vi "Auto Mode Alternate 2.vi"(1 "error in (no error)":errorcluster) -> ()   [LabVIEW 2017]
uses:
  <vilib>/Rock Robotics/WPI/Utilities/WPI_GetSetVariantRefNum.vi
  <vilib>/Rock Robotics/Network Tables/NT Write Numeric Array.vi
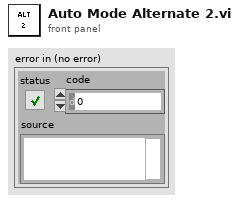
[diagram p1: front panel]
types:
  T1 = typedef "WPI_RobotDriveDevRef.ctl" = cluster{"DevStatus":errorcluster, "Motors[]":T2[], "Square Inputs":bool, "Max Output":dbl}
  T2 = typedef "WPI_MotorControlDeviceRef.ctl" = cluster{"DeviceStatus":errorcluster, "Type":T3, "PWM":cluster{"PWM Channel":T4, "DeadBand":T5}, "CAN":cluster{"Device Number":u8, "SetOutput VI Ref":variant, "GetOutput VI Ref":variant, "Enable VI Ref":variant, "Disable VI Ref":variant, "Data":variant}, "Invert":bool, "DIO PWM":cluster{"PWM \"Enable\" Channel":T4, "DIOChannel":T6, "PWM Rate":dbl}}
  T3 = typedef "WPI_MotorControlType.ctl" = enum16{"PWM", "CAN", "DIO PWM"}
  T4 = typedef "FPGA_DIOPWMChannel.ctl" = enum8{"PWM 0", "PWM 1", "PWM 2", "PWM 3", "PWM 4", "PWM 5", "PWM 6", "PWM 7", "PWM 8", "PWM 9", "PWM MXP 0", "PWM MXP 1", "PWM MXP 2", "PWM MXP 3", "PWM MXP 4", "PWM MXP 5", "PWM MXP 6", "PWM MXP 7", "PWM MXP 8", "PWM MXP 9", "Invalid"}
  T5 = typedef "WPI_PWMDeadband.ctl" = cluster{"Name":string, "maxPositivePwm":i32, "minPositivePwm":i32, "centerPwm":i32, "maxNegativePwm":i32, "minNegativePwm":i32, "angularRange":u16}
  T6 = typedef "FPGA_DIOChannel.ctl" = enum8{"DIO 0", "DIO 1", "DIO 2", "DIO 3", "DIO 4", "DIO 5", "DIO 6", "DIO 7", "DIO 8", "DIO 9", "DIO MXP 0", "DIO MXP 1", "DIO MXP 2", "DIO MXP 3", "DIO MXP 4", "DIO MXP 5", "DIO MXP 6", "DIO MXP 7", "DIO MXP 8", "DIO MXP 9", "DIO MXP 10", "DIO MXP 11", "DIO MXP 12", "DIO MXP 13", "DIO MXP 14", "DIO MXP 15", "SPI Port CS1", "SPI Port CS2", "SPI Port CS3", "SPI Port MISO", "SPI Port MOSI", "Invalid"}
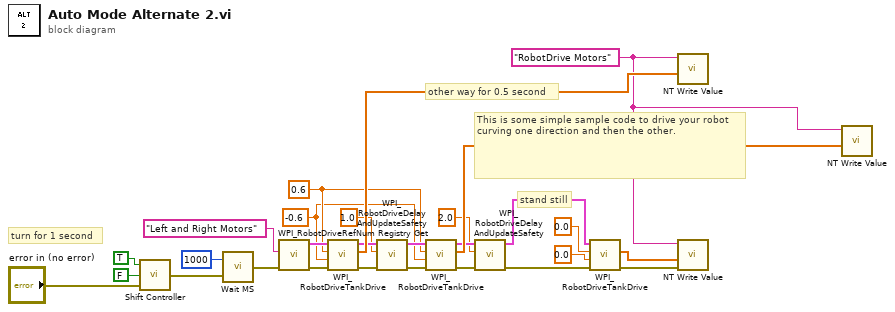
[diagram p0: block diagram]
diagram:
  w1 = -0.6
  w2 = 0.6
  w18 = "RobotDrive Motors" ("Name")
  # "stand still"
  # "other way for 0.5 second"
  # "turn for 1 second"
  # "This is some simple sample code to drive your robot curving one direction and then the other."
  n1 = call "Shift Controller.vi"("error in"="error in (no error)", "Right Trigger"=FALSE, "Left Trigger"=TRUE) -> ("error out"=w4:errorcluster)
  n2 = call "Wait MS.vi"("error in"=w4, "milliseconds to wait"=u32 1000) -> ("error out"=w3:errorcluster)
  n3 = call <vilib>:"WPI_RobotDriveRefNum Registry Get.vi"("error in (no error)"=w3, "refnum name"="Left and Right Motors") -> ("error out"=w23:errorcluster, "RobotDriveDevRef"=w6:T1)  [unwired: 8 out]
  n4 = call <vilib>:"WPI_RobotDriveTankDrive.vi"("error in (no error)"=w23, "Right axis value"=w1, "Left axis value"=w2, "RobotDriveDevRef"=w6) -> ("error out"=w24:errorcluster, "Motor Values"=w19:dbl[], "RobotDriveDevRef"=w13:T1)  [unwired: 5 in]
  n5 = call <vilib>:"WPI_RobotDriveDelayAndUpdateSafety.vi"("error in (no error)"=w24, "Delay (s)"=1.0, "RobotDriveDevRef"=w13) -> ("error out"=w25:errorcluster, "RobotDriveDevRef 2"=w12:T1)  [unwired: 7 in]
  n6 = call <vilib>:"WPI_RobotDriveTankDrive.vi"("error in (no error)"=w25, "Right axis value"=w1, "Left axis value"=w2, "RobotDriveDevRef"=w12) -> ("error out"=w26:errorcluster, "Motor Values"=w17:dbl[], "RobotDriveDevRef"=w11:T1)  [unwired: 5 in]
  n7 = call <vilib>:"WPI_RobotDriveDelayAndUpdateSafety.vi"("error in (no error)"=w26, "Delay (s)"=2.0, "RobotDriveDevRef"=w11) -> ("error out"=w27:errorcluster, "RobotDriveDevRef 2"=w10:T1)  [unwired: 7 in]
  n8 = call <vilib>:"WPI_RobotDriveTankDrive.vi"("error in (no error)"=w27, "Right axis value"=0.0 ("X axis value"), "Left axis value"=0.0 ("X axis value"), "RobotDriveDevRef"=w10) -> ("error out"=w28:errorcluster, "Motor Values"=w16:dbl[])  [unwired: 5 in, 1 out]
  n9 = call-poly <vilib>:"NT Write Value.vi"("Numeric Array"=w19, "Name"=w18) -> ()  [unwired: 9 in, 1 out]
  n10 = call-poly <vilib>:"NT Write Value.vi"("error in"=w28, "Numeric Array"=w16, "Name"=w18) -> ()  [unwired: 8 in, 1 out]
  n11 = call-poly <vilib>:"NT Write Value.vi"("Numeric Array"=w17, "Name"=w18) -> ()  [unwired: 9 in, 1 out]
